vi "ERRMSG.VI"(0 "ErrCode":i32) -> (1 "ErrMsg":string, 2 "ErrCode (Out)":i32)   [LabVIEW 2019, in "DAQ_Engine.lvclass"]
doc: "Developed by Kevin Thompson\nkevin@thompsonengineering.net\n\nCopyright 2020\nThompson Engineering, LLC\nReturns the error message associated with an error code."
uses:
  DAQ_Engine.lvclass
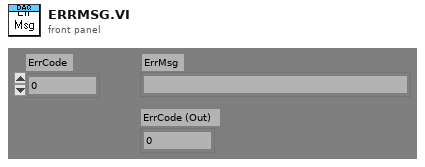
[diagram p1: front panel]
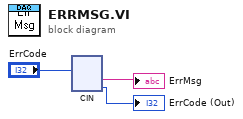
[diagram p0: block diagram]
diagram:
  n1 = cin("ErrCode") -> (→"ErrMsg":string, →"ErrCode (Out)":i32)  [unwired: 3 in]
